vi "Plot_Lineouts.vi"(0 "scale_end":dbl=1.0 format="%0.2f", 1 "end":dbl=1.0 format="%0.2f", 2 "scale_start":dbl=1.0 format="%0.2f", 3 "start":dbl format="%0.2f", 5 "transpose?":bool, 6 "lineouts":dbl[][](array[numeric]), 7 "ref":refnum<vi>) -> ()   [LabVIEW 2010]
uses:
  <vilib>/Analysis/1siggen.llb/Ramp Pattern by Samples.vi
  <vilib>/Analysis/NI_AALBase.lvlib
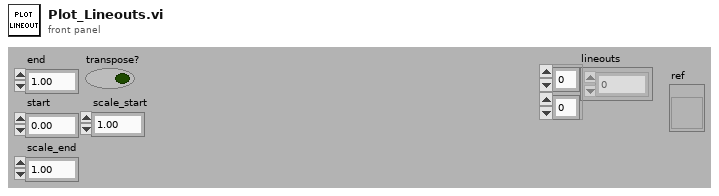
[diagram p1: front panel]
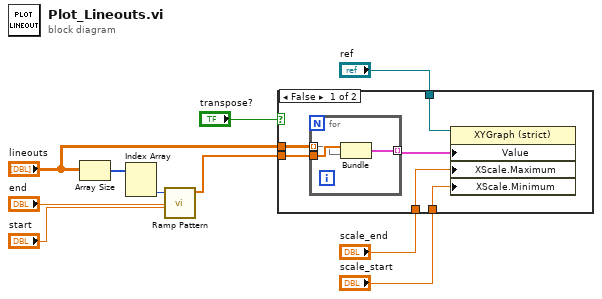
[diagram p0: block diagram]
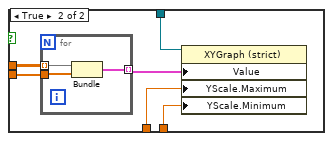
[diagram p2: hidden frame]
diagram:
  n1 = Array Size(array="lineouts") -> (size(s)=w10:i32[])
  n2 = Index Array(array=w10) -> (element #2=w9:i32)  [unwired: 2 in, 1 out]
  n3 = call-poly <vilib>:"Ramp Pattern.vi"("start"="start", "end"="end", "samples"=w9) -> ("Ramp Pattern"=w5:dbl[])  [unwired: 7 in, 1 out]
  n4 = case shown="False" "transpose?" {
    tunnel: "lineouts" -> [w16 w25]
    tunnel: w5 -> [w15 w24]
    tunnel: "scale_end" -> [w13 w22]
    tunnel: "scale_start" -> [w12 w21]
    tunnel: "ref" -> [w11 w20]
    frame False {
      n5 = for {
        tunnel: w16 -> [w18] mode=indexing
        tunnel: w15 -> [w19]
        tunnel: [w17] -> w14 mode=indexing
        n6 = Bundle("Ramp Pattern"=w19, "lineouts"=w18) -> (w17:cluster{"Ramp Pattern":dbl[], "lineouts":dbl[]})  [unwired: 1 in]
      }
      n7 = property class="XYGraph (strict)"(reference=w11, "Value"=w14, "XScale.Maximum"=w13, "XScale.Minimum"=w12) -> ()  [unwired: 1 in, 2 out]
    }
    frame True {
      n8 = for {
        tunnel: w25 -> [w27] mode=indexing
        tunnel: w24 -> [w26]
        tunnel: [w28] -> w23 mode=indexing
        n9 = Bundle("lineouts"=w27, "Ramp Pattern"=w26) -> (w28:cluster{"lineouts":dbl[], "Ramp Pattern":dbl[]})  [unwired: 1 in]
      }
      n10 = property class="XYGraph (strict)"(reference=w20, "Value"=w23, "YScale.Maximum"=w22, "YScale.Minimum"=w21) -> ()  [unwired: 1 in, 2 out]
    }
  }
